vi "PXI-Update AI.vi"(0 "AI Tasks":T1[](array[typedef]), 5 "Skip samples":i32, 11 "error in (no error)":errorcluster, 12 "cycle":i32) -> (15 "error out":errorcluster)   [LabVIEW 2020]
uses:
  Type Defs/Task Struct.ctl
  Type Defs/PXI-DO Signal Bank Action.ctl
  PXI Globals.vi
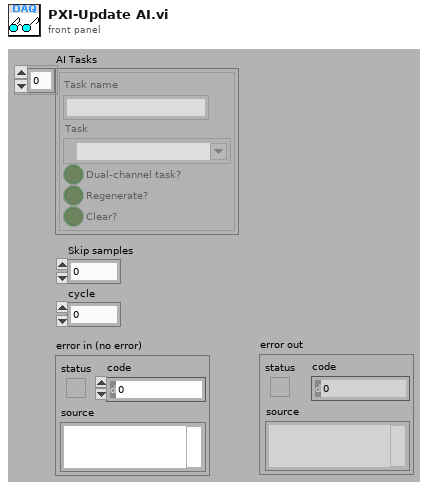
[diagram p1: front panel]
types:
  T1 = typedef "Task Struct.ctl" = cluster{"Task name":string, "Task":refnum<k21>, "Dual-channel task?":bool, "Regenerate?":bool, "Clear?":bool}
  T2 = typedef "PXI-DO Signal Bank Action.ctl" = enum16{"Clear", "Write", "Read"}
  T3 = typedef "PXI-AI Transfer Mode.ctl" = enum16{"Queue", "Data Bank", "No Transfer"}
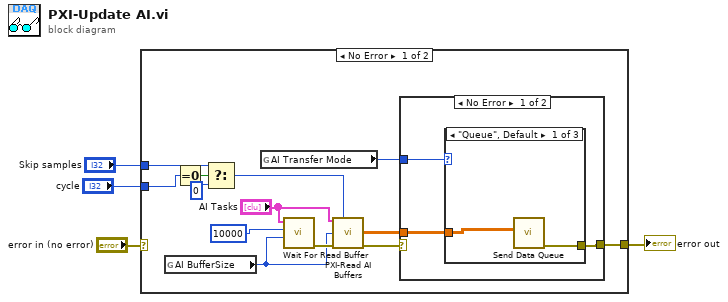
[diagram p0: block diagram]
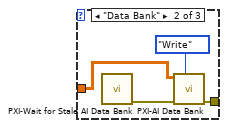
[diagram p2: hidden frame]
diagram:
  n1 = case shown="No Error" "error in (no error)" {
    selector: "error in (no error)" -> [_ w28]
    tunnel: "Skip samples" -> [w13 _]
    tunnel: "cycle" -> [w12 _]
    tunnel: [w10 w28] -> w2
    frame No Error {
      n2 = global read "PXI Globals.vi" "AI BufferSize"() -> (w6:i32)
      n3 = Equal To 0?(x=w12) -> (x = 0?=w15:bool)
      n4 = Select(t=w13, s=w15, f=0) -> (s? t:f=w16:i32)
      n5 = global read "PXI Globals.vi" "AI Transfer Mode"() -> (w5:T3)
      n6 = call "Wait For Read Buffer.vi"("BufferSize"=w6, "timeout (ms)"=10000 ("BufferSize"), "AI Tasks"="AI Tasks") -> ("error out"=w9:errorcluster)  [unwired: 8 in]
      n7 = call "PXI-Read AI Buffers.vi"("AI Tasks"="AI Tasks", "Samples to skip"=w16, "Samples per channel"=w6, "error in (no error)"=w9) -> ("AI Waveforms"=w14:dbl[][], "error out"=w11:errorcluster)  [unwired: 9 in, 1 out]
      n8 = case shown="No Error" w11 {
        selector: w11 -> [_ w27]
        tunnel: w14 -> [w20 _]
        tunnel: [w19 w27] -> w10
        tunnel: w5 -> [w18 _]
        frame No Error {
          n9 = case shown="\"Queue\", Default" w18 {
            tunnel: w20 -> [w22 w25 _]
            tunnel: [w21 w24 _] -> w19
            frame "Queue", Default {
              n10 = call "Send Data Queue.vi"("AI Waveforms"=w22) -> ("error out"=w21:errorcluster)  [unwired: 6 in]
            }
            frame "Data Bank" {
              n11 = call "PXI-Wait for Stale AI Data Bank.vi"() -> ("error out"=w26:errorcluster)  [unwired: 11 in]
              n12 = call "PXI-AI Data Bank.vi"("Action"=PXI-DO_Signal_Bank_Action."Write", "error in (no error)"=w26, "Data In"=w25) -> ("error out"=w24:errorcluster)  [unwired: 7 in, 1 out]
            }
            frame "No Transfer" {
            }
          }
        }
        frame Error {
        }
      }
    }
    frame Error {
    }
  }
  "error out" <- w2
